vi "Globals.vi"() -> ()   [LabVIEW 2014, in "LAVA TIFF File Reader.lvlib"]
uses:
  LAVA TIFF File Reader.lvlib
panel:
  in  "Litt/BigEnd":bool
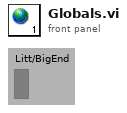
[diagram p1: front panel]
diagram:
